vi "checkin.vi"(8 "error in (no error)":errorcluster, 11 "GeneralAnalyser in":refnum<class "GenericAnalyser.lvclass">) -> (0 "error out":errorcluster, 3 "GeneralAnalyser out":refnum<class "GenericAnalyser.lvclass">)   [LabVIEW 2010, in "GenericAnalyser.lvclass"]
uses:
  GenericAnalyser.lvclass
  common/classes/GenericToplevelComponent/GenericToplevelComponent/GenericToplevelComponent.lvclass
  class_data.vi
  common/classes/GenericComponent/GenericComponent/GenericComponent.lvclass
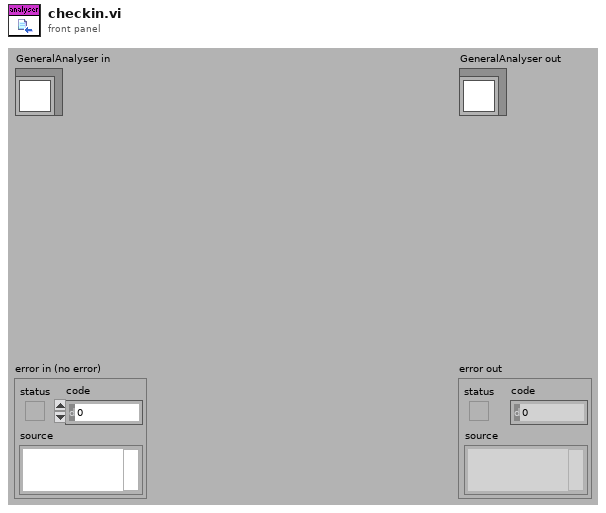
[diagram p1: front panel]
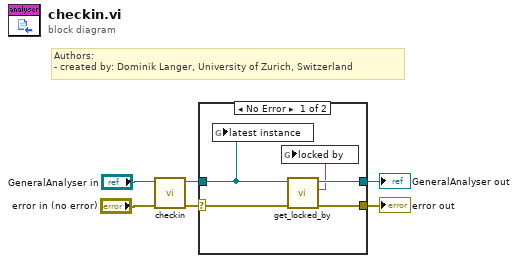
[diagram p0: block diagram]
diagram:
  # "Authors: \n- created by: Dominik Langer, University of Zurich, Switzerland"
  n1 = call-parent "checkin.vi"("error in (no error)"="error in (no error)", "GenericPlugin in"="GeneralAnalyser in") -> ("error out"=w3:errorcluster, "GenericPlugin out"=w1:refnum<class "GenericAnalyser.lvclass">)  [unwired: 8 in]
  n2 = case shown="No Error" w3 {
    selector: w3 -> [w7 w13]
    tunnel: [w11 w13] -> w6
    tunnel: [w10 w12] -> w5
    tunnel: w1 -> [w8 w12]
    frame No Error {
      n3 = global write "class_data.vi" "latest instance"(w8) -> ()
      n4 = call "get_locked_by.vi"("error in (no error)"=w7, "GenericPlugin.lvclass in"=w8) -> ("error out"=w11:errorcluster, "locked by"=w9:string, "GenericPlugin.lvclass out"=w10:refnum<class "GenericAnalyser.lvclass">)  [unwired: 7 out]
      n5 = global write "class_data.vi" "locked by"(w9) -> ()
    }
    frame Error {
    }
  }
  "error out" <- w6
  "GeneralAnalyser out" <- w5
